vi "Get Group.vi"(10 "id":string, 11 "DSF Configuration in":T4) -> (0 "exists?":bool, 2 "info":T1, 3 "DSF Configuration out":T4, 4 "index":i32)   [LabVIEW 2017, in "Data Sharing Framework Configuration.lvlib"]
uses:
  Data Sharing Framework Configuration.lvlib
  Controls/Session/DSF Config Data.ctl
  Controls/DSF File Format/Internal.DSF Configuration.ctl
  Public/Controls/DSF Version Info.ctl
  Controls/DSF File Format/Internal.DSF Plugin with ID.ctl
  Controls/DSF File Format/Internal.DSF Plugin Info.ctl
  Public/Controls/DSF Timing Info.ctl
  Controls/DSF File Format/Internal.DSF Group with ID.ctl
  Controls/DSF File Format/Internal.DSF Group Info.ctl
  Controls/DSF File Format/Internal.DSF Transfer with ID.ctl
  Controls/DSF File Format/Internal.DSF Transfer Info.ctl
  Controls/DSF File Format/Internal.DSF Channel with ID.ctl
  Controls/DSF File Format/Internal.DSF Channel Info.ctl
  Controls/DSF File Format/Internal.DSF Settings with ID.ctl
  Controls/DSF File Format/Internal.DSF Settings Info.ctl
  Public/Controls/DSF Group Info.ctl
  Public/Controls/DSF Direction.ctl
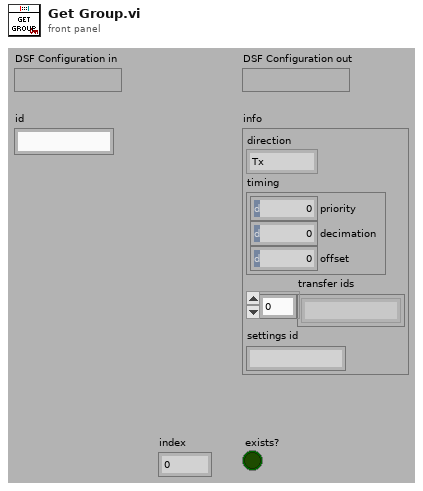
[diagram p1: front panel]
types:
  T1 = typedef "Data Sharing Framework Configuration.lvlib/DSF Group Info.ctl" = cluster{"direction":T2, "timing":T3, "transfer ids":string[], "settings id":string}
  T2 = typedef "Data Sharing Framework Configuration.lvlib/DSF Direction.ctl" = enum8{"Tx", "Rx"}
  T3 = typedef "Data Sharing Framework Configuration.lvlib/DSF Timing Info.ctl" = cluster{"priority":u64, "decimation":u64, "offset":u64}
  T4 = typedef "Data Sharing Framework Configuration.lvlib/DSF Config Data.ctl" = cluster{"dsf configuration":T5, "path":path, "dirty":bool}
  T5 = typedef "Data Sharing Framework Configuration.lvlib/Internal.DSF Configuration.ctl" = cluster{"dsfversion":T6, "version":T6, "plugins":T7[], "groups":T9[], "transfers":T11[], "channels":T13[], "settings":T15[]}
  T6 = typedef "Data Sharing Framework Configuration.lvlib/DSF Version Info.ctl" = cluster{"major":u32, "minor":u32, "fix":u32, "build":string}
  T7 = typedef "Data Sharing Framework Configuration.lvlib/Internal.DSF Plugin with ID.ctl" = cluster{"id":string, "values":T8}
  T8 = typedef "Data Sharing Framework Configuration.lvlib/Internal.DSF Plugin Info.ctl" = cluster{"type":string, "timing":T3, "group ids":string[], "settings id":string}
  T9 = typedef "Data Sharing Framework Configuration.lvlib/Internal.DSF Group with ID.ctl" = cluster{"id":string, "values":T10}
  T10 = typedef "Data Sharing Framework Configuration.lvlib/Internal.DSF Group Info.ctl" = cluster{"direction":i32, "timing":T3, "transfer ids":string[], "settings id":string}
  T11 = typedef "Data Sharing Framework Configuration.lvlib/Internal.DSF Transfer with ID.ctl" = cluster{"id":string, "values":T12}
  T12 = typedef "Data Sharing Framework Configuration.lvlib/Internal.DSF Transfer Info.ctl" = cluster{"byte order":i32, "channel ids":string[], "settings id":string}
  T13 = typedef "Data Sharing Framework Configuration.lvlib/Internal.DSF Channel with ID.ctl" = cluster{"id":string, "values":T14}
  T14 = typedef "Data Sharing Framework Configuration.lvlib/Internal.DSF Channel Info.ctl" = cluster{"count":u64, "buffer offset":u64, "data type":i32, "settings id":string}
  T15 = typedef "Data Sharing Framework Configuration.lvlib/Internal.DSF Settings with ID.ctl" = cluster{"id":string, "values":T16}
  T16 = typedef "Data Sharing Framework Configuration.lvlib/Internal.DSF Settings Info.ctl" = cluster{"key":string, "value":string}[]
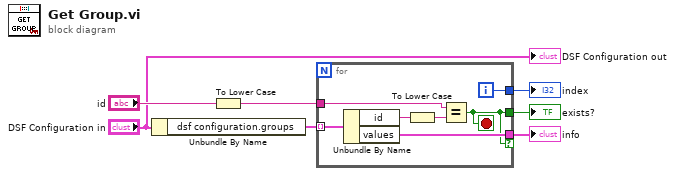
[diagram p0: block diagram]
diagram:
  n1 = Unbundle By Name("DSF Configuration in") -> ("dsf configuration.groups"=w7:T9[])
  n2 = To Lower Case(string="id") -> (all lower case string=w6:string)
  n3 = for {
    tunnel: w7 -> [w14] mode=indexing
    tunnel: w6 -> [w11]
    tunnel: [w8] -> w2
    tunnel: [w10] -> w1
    tunnel: [w9] -> w3 if=w8
    i -> [w10]
    stop <- w8 stop-if-true
    n4 = Unbundle By Name(w14) -> ("id"=w12:string, "values"=w9:T10)
    n5 = To Lower Case(string=w12) -> (all lower case string=w13:string)
    n6 = Equal?(x=w11, y=w13) -> (x = y?=w8:bool)
  }
  "index" <- w1
  "exists?" <- w2
  "info" <- w3
  "DSF Configuration out" <- "DSF Configuration in"
